vi "Apply Archive Configuration.vi"(8 "error in (no error)":errorcluster, 10 "Timer Handler":T1, 11 "System Configuration":T2) -> (0 "error out":errorcluster, 3 "Succeed?":bool)   [LabVIEW 2024]
doc: "Applies archive configurations."
uses:
  Controls/Server/System Configuration.ctl
  Controls/Server/Subsystem Configuration.ctl
  Timer/Timer Handler.ctl
  Globals/Global - Server.vi
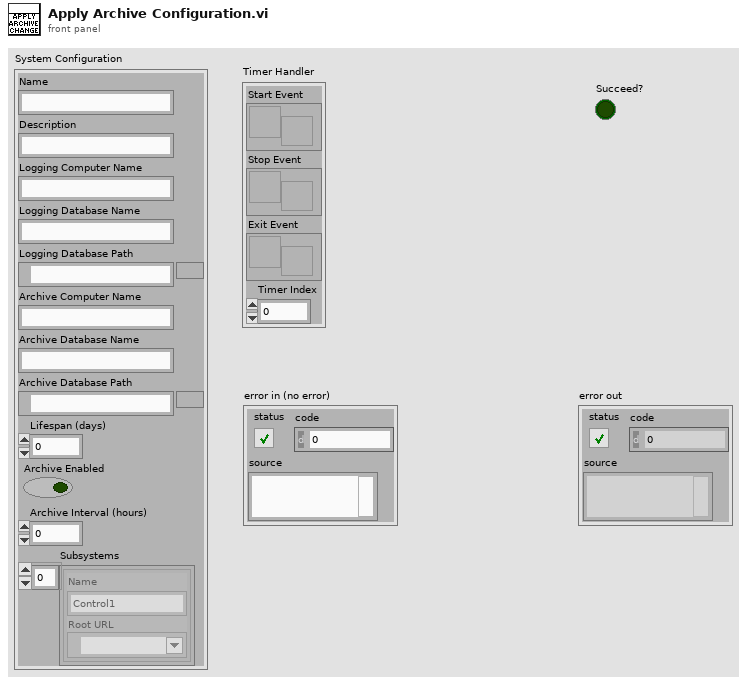
[diagram p1: front panel]
types:
  T1 = typedef "Timer Handler.ctl" = cluster{"Start Event":refnum<user-event>, "Stop Event":refnum<user-event>, "Exit Event":refnum<user-event>, "Timer Index":u32}
  T2 = typedef "System Configuration.ctl" = cluster{"Name":string, "Description":string, "Logging Computer Name":string, "Logging Database Name":string, "Logging Database Path":path, "Archive Computer Name":string, "Archive Database Name":string, "Archive Database Path":path, "Lifespan (days)":u32, "Archive Enabled":bool, "Archive Interval (hours)":u32, "Subsystems":T3[]}
  T3 = typedef "Subsystem Configuration.ctl" = cluster{"Name":string, "Root URL":refnum<k21>}
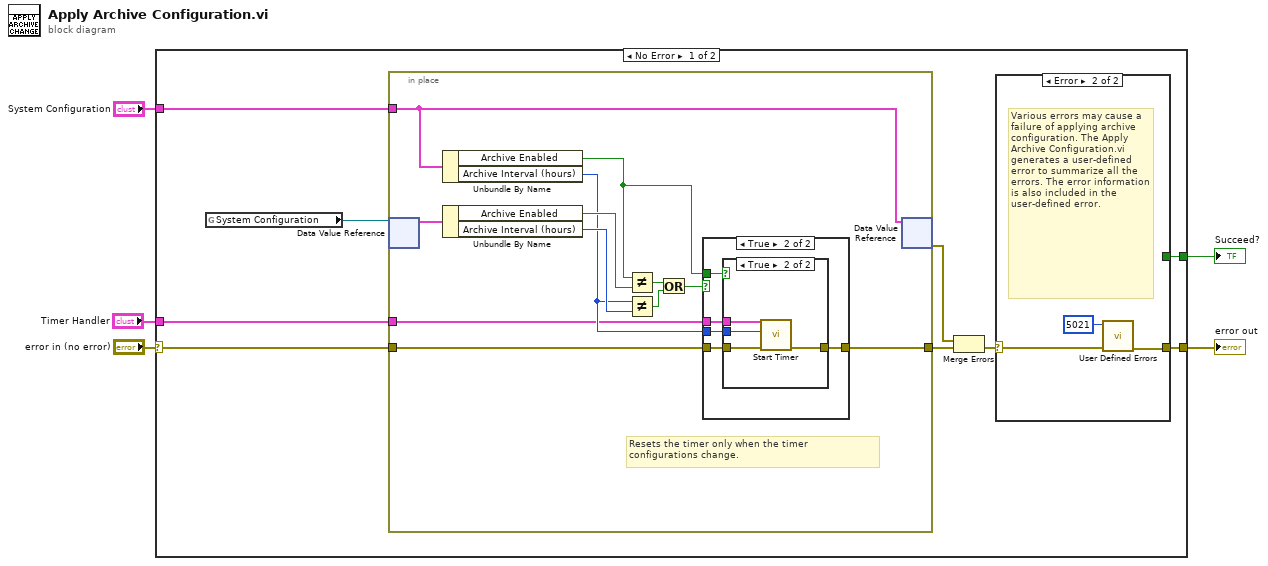
[diagram p0: block diagram]
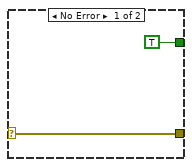
[diagram p2: hidden frame]
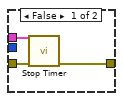
[diagram p4: hidden frame]
diagram:
  n1 = case shown="No Error" "error in (no error)" {
    selector: "error in (no error)" -> [w14 w45]
    tunnel: [w7 w45] -> w4
    tunnel: "System Configuration" -> [w10 _]
    tunnel: "Timer Handler" -> [w9 _]
    tunnel: [w6 _] -> w1
    frame No Error {
      n2 = global read "Global - Server.vi" "System Configuration"() -> (w13:refnum<data-value>)
      n3 = in-place {
        in-place-border: w10 -> [w22]
        in-place-border: w14 -> [w24]
        in-place-border: [w20] -> w12
        in-place-border: w9 -> [w21]
        # "Resets the timer only when the timer configurations change."
        n4 = in-place-dvr #1(w13) -> (w23:T2)  [unwired: 1 out]
        n5 = Unbundle By Name(w22) -> ("Archive Enabled"=w31:bool, "Archive Interval (hours)"=w28:u32)
        n6 = Unbundle By Name(w23) -> ("Archive Enabled"=w30:bool, "Archive Interval (hours)"=w29:u32)
        n7 = Not Equal?(x=w31, y=w30) -> (x != y?=w27:bool)
        n8 = Not Equal?(x=w28, y=w29) -> (x != y?=w26:bool)
        n9 = Or(x=w27, y=w26) -> (x .or. y?=w25:bool)
        n10 = case shown="True" w25 {
          tunnel: w28 -> [_ w37]
          tunnel: w31 -> [_ w36]
          tunnel: w24 -> [w32 w35]
          tunnel: [w32 w34] -> w20
          tunnel: w21 -> [_ w33]
          frame False {
          }
          frame True {
            n11 = case shown="True" w36 {
              tunnel: w33 -> [w40 w44]
              tunnel: w37 -> [_ w43]
              tunnel: [w39 w42] -> w34
              tunnel: w35 -> [w38 w41]
              frame False {
                n12 = call "Stop Timer.vi"("error in (no error)"=w38, "Timer Handler"=w40) -> ("error out"=w39:errorcluster)  [unwired: 9 in]
              }
              frame True {
                n13 = call "Start Timer.vi"("error in (no error)"=w41, "Timer Interval (hours)"=w43, "Timer Handler"=w44) -> ("error out"=w42:errorcluster)  [unwired: 8 in]
              }
            }
          }
        }
        n14 = in-place-dvr #1(w22) -> (w11:errorcluster)  [unwired: 1 out]
      }
      n15 = Merge Errors(w11, w12) -> (w8:errorcluster)
      n16 = case shown="Error" w8 {
        selector: w8 -> [w16 w19]
        tunnel: [w16 w18] -> w7
        tunnel: [TRUE ("Succeed?") _] -> w6
        frame No Error {
        }
        frame Error {
          # "Various errors may cause a failure of applying archive configuration. The Apply Archive Configuration.vi generates a user-defined error to summarize all the errors. The error information is also included in the user-defined error."
          n17 = call "User Defined Errors.vi"("error in (no error)"=w19, "Error Code (0)"=5021 ("error code (0)")) -> ("error out"=w18:errorcluster)  [unwired: 9 in]
        }
      }
    }
    frame Error {
    }
  }
  "error out" <- w4
  "Succeed?" <- w1
